vi "Msg Remain.vi"(10 "Remaining Elements":refnum<class "Msg.lvclass">[](array[class]), 11 "Process in":refnum<class "Process.lvclass">) -> ()   [LabVIEW 2021, in "Process.lvlib" / "Process.lvclass"]
uses:
  Process.lvclass
  AAM/AAM/Msg/Msg.lvclass
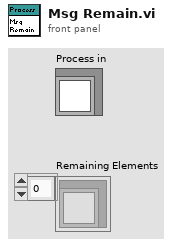
[diagram p1: front panel]
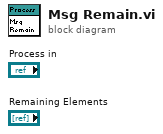
[diagram p0: block diagram]
diagram:
